vi "HELMET.vi"() -> ()   [LabVIEW 2022 SP3]
uses:
  <vilib>/Instr/_visa.llb/VISA Configure Serial Port (Instr).vi
panel:
  out "substring 4":string
  out "substring 3":string
  out "substring 2":string
  out "substring":string
  in  "milliseconds to wait":u32
  in  "stop":bool
  out "read buffer":string
  in  "byte count":u32
  in  "VISA resource name":refnum<visa-resource-name>
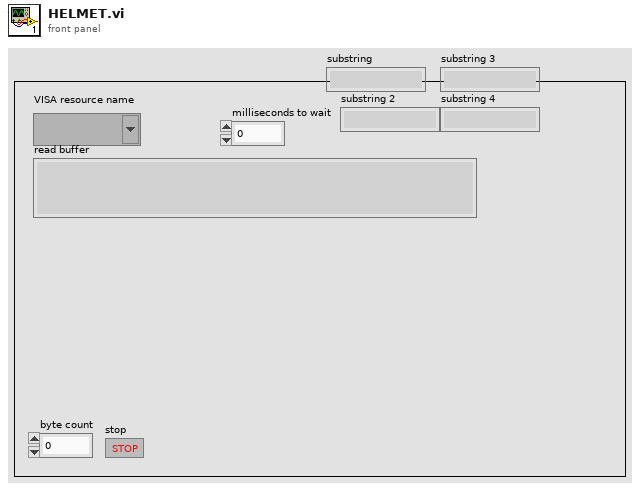
[diagram p1: front panel]
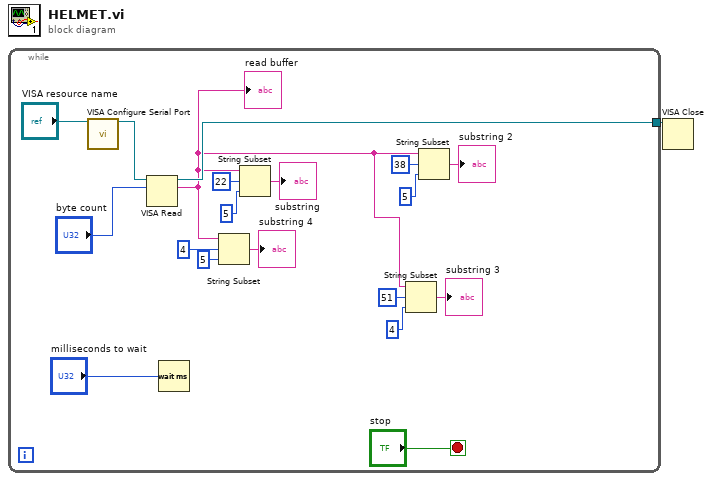
[diagram p0: block diagram]
diagram:
  n1 = while {
    tunnel: [w17] -> w1
    stop <- "stop" stop-if-true
    n2 = call-poly "VISA Configure Serial Port"("VISA resource name"="VISA resource name") -> ("VISA resource name out"=w19:refnum<visa-resource-name>)  [unwired: 13 in, 1 out]
    n3 = VISA Read(VISA resource name=w19, byte count="byte count") -> (VISA resource name out=w17:refnum<visa-resource-name>, read buffer=w6:string)  [unwired: 1 in, 2 out]
    "read buffer" <- w6
    n4 = Wait (ms)(milliseconds to wait="milliseconds to wait") -> ()  [unwired: 1 out]
    n5 = String Subset(string=w6, offset (0)=4, length (rest)=5 ("length (rest)")) -> (substring=→"substring 4":string)
    n6 = String Subset(string=w6, offset (0)=22, length (rest)=5 ("length (rest)")) -> (substring=→"substring":string)
    n7 = String Subset(string=w6, offset (0)=51, length (rest)=4 ("length (rest)")) -> (substring=→"substring 3":string)
    n8 = String Subset(string=w6, offset (0)=38, length (rest)=5 ("length (rest)")) -> (substring=→"substring 2":string)
  }
  n9 = VISA Close(VISA resource name=w1) -> ()  [unwired: 1 in, 1 out]
